vi "Read_Gripper_State.vi"(0 "error in":errorcluster, 2 "Side":T2, 3 "node":string) -> (1 "error out":errorcluster, 4 "EndEffectorState":T1)   [LabVIEW 2012]
doc: "Returns information from subscription to /sdk/robot/limb/<limb>/accessory/gripper/state"
uses:
  <userlib>/rosforlv/ROS/Code/SubVIs/BaxterSide.ctl
  <userlib>/rosforlv/ROS/Code/Console/Servers/ServerSubs/TopicDef.ctl
  <userlib>/rosforlv/ROS/Code/SubVIs/_ROSDirection.ctl
panel:
  out "Reply":string
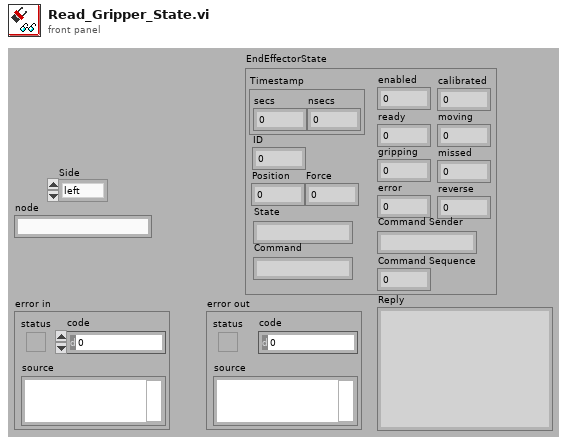
[diagram p1: front panel]
types:
  T1 = cluster{"Timestamp":cluster{"secs":i32, "nsecs":i32}, "ID":u32, "enabled":u8, "calibrated":u8, "ready":u8, "moving":u8, "gripping":u8, "missed":u8, "error":u8, "reverse":u8, "Position":sgl, "Force":sgl, "State":string, "Command":string, "Command Sender":string, "Command Sequence":u32}
  T2 = typedef "BaxterSide.ctl" = enum16{"left", "right"}
  T3 = typedef "TopicDef.ctl" = cluster{"Topic":string, "Type":string, "Action":T4, "Update (ms)":u16, "write queue":u16}
  T4 = typedef "_ROSDirection.ctl" = enum16{"Node", "Publisher", "Subscriber", "Service Client"}
  T5 = typedef "_ROSControl.ctl" = cluster{"topic port":u16, "Node":string, "topic":string, "type":string, "node port":u32, "error ":errorcluster, "Direction":T4, "APIs":string[], "Update (ms)":u16, "write queue":u16}
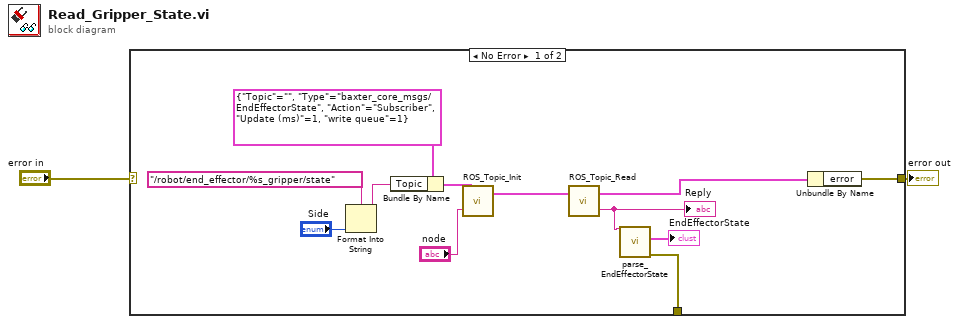
[diagram p0: block diagram]
diagram:
  n1 = case shown="No Error" "error in" {
    selector: "error in" -> [_ w15]
    tunnel: [w14 w15] -> w2
    tunnel: [w3 _] -> _
    frame No Error {
      n2 = Format Into String(format string="/robot/end_effector/%s_gripper/state" ("Topic"), "Side") -> (resulting string=w9:string)  [unwired: 2 in, 1 out]
      n3 = Bundle By Name(cluster=T3 {"Topic"="", "Type"="baxter_core_msgs/EndEffectorState", "Action"=enum."Subscriber", "Update (ms)"=1, "write queue"=1} ("Definitions"), "Topic"=w9) -> (w6:T3)
      n4 = call <userlib>:"ROS_Topic_Init.vi"("node"="node", "Definitions"=w6) -> ("ROS out"=w12:T5)  [unwired: 1 in]
      n5 = call <userlib>:"ROS_Topic_Read.vi"("ROS in"=w12) -> ("Reply"=w5:string, "ROS out"=w11:T5)  [unwired: 1 in]
      "Reply" <- w5
      n6 = call <userlib>:"parse_EndEffectorState.vi"("msg in"=w5) -> ("error out"=w3:errorcluster, "EndEffectorState"=→"EndEffectorState":T1)  [unwired: 4 in, 1 out]
      n7 = Unbundle By Name(w11) -> ("error"=w14:errorcluster)
    }
    frame Error {
    }
  }
  "error out" <- w2
